vi "PathFinder.vi"(7 "Cost":T3(c390), 8 "TotalCost":u64, 9 "Direction":T1, 11 "AnalysePosition":T2) -> (2 "Directions":T1[](array[typedef]), 3 "Positions":T2[](array[typedef]))   [LabVIEW 2023, in "2024_16.lvclass"]
uses:
  2024_16.lvclass
  Common/AOC_XY(I32).ctl
  Common/AOC_Direction.ctl
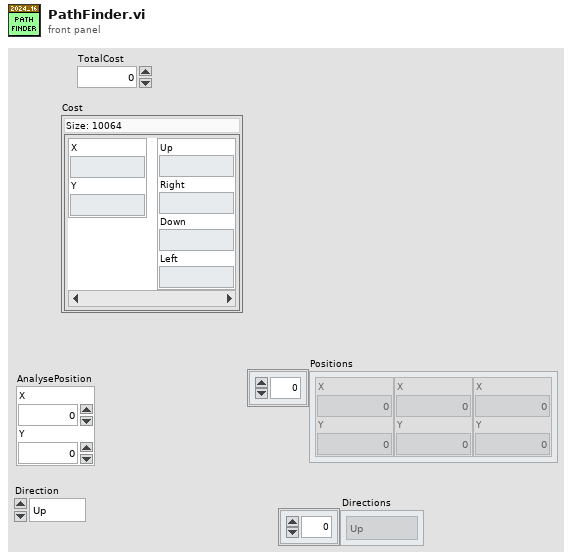
[diagram p1: front panel]
types:
  T1 = typedef "AOC_Direction.ctl" = enum16{"Up", "Right", "Down", "Left"}
  T2 = typedef "AOC_XY(I32).ctl" = cluster{"X":i32, "Y":i32}
  T3 = map{T2, cluster{"Up":u64, "Right":u64, "Down":u64, "Left":u64}}
  T4 = cluster{"Up":u64, "Right":u64, "Down":u64, "Left":u64}
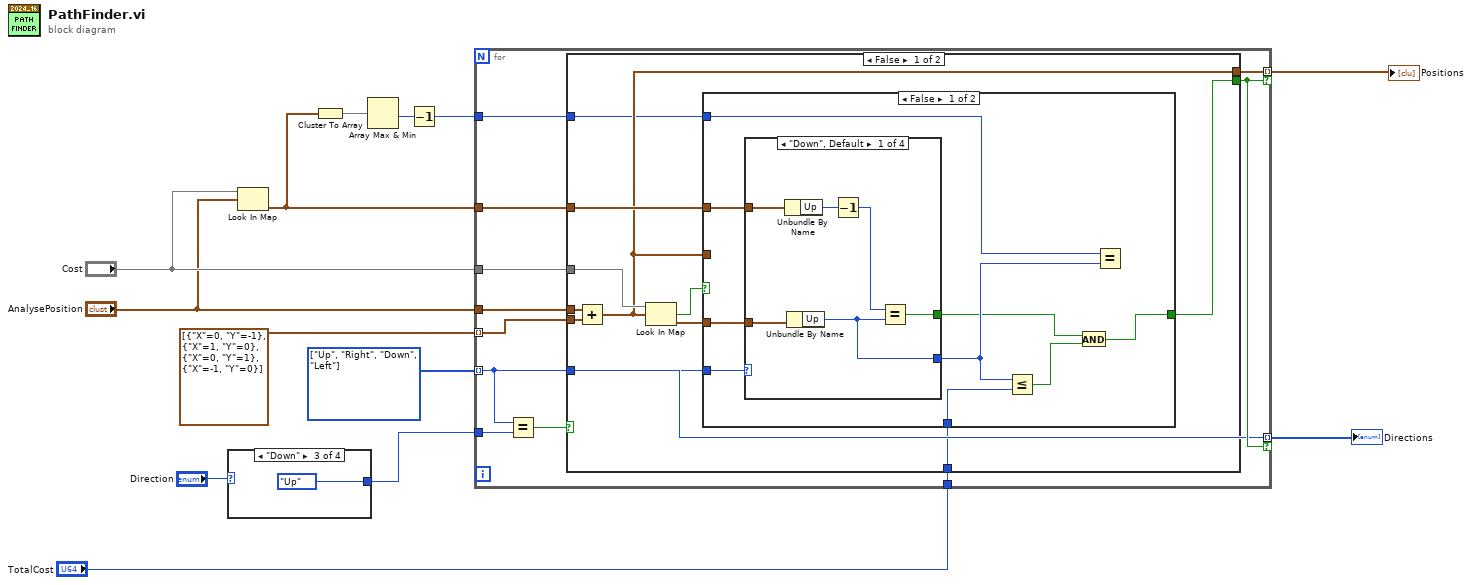
[diagram p0: block diagram]
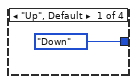
[diagram p2: hidden frame]
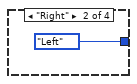
[diagram p3: hidden frame]
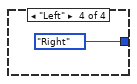
[diagram p4: hidden frame]
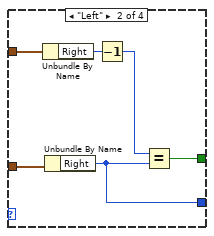
[diagram p5: hidden frame]
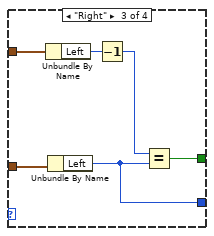
[diagram p6: hidden frame]
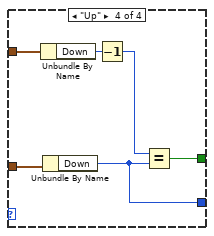
[diagram p7: hidden frame]
diagram:
  w10 = T1[] [enum."Up", enum."Right", enum."Down", enum."Left"] items=["Up", "Right", "Down", "Left"]
  n1 = case shown="\"Down\"" "Direction" {
    tunnel: [AOC_Direction."Down" ("Enum") AOC_Direction."Left" ("Enum") AOC_Direction."Up" ("Enum") AOC_Direction."Right" ("Enum")] -> w6
    frame "Up", Default {
    }
    frame "Right" {
    }
    frame "Down" {
    }
    frame "Left" {
    }
  }
  n2 = Look In Map(map="Cost", key="AnalysePosition") -> (value=w5:T4)  [unwired: 1 in, 1 out]
  n3 = Cluster To Array(cluster=w5) -> (array=w4:u64[])
  n4 = Array Max & Min(array=w4) -> (min value=w3:u64)  [unwired: 3 out]
  n5 = Decrement(x=w3) -> (x-1=w2:u64)
  n6 = for {
    tunnel: cluster{"X":i32, "Y":i32}[] [{"X"=0, "Y"=-1}, {"X"=1, "Y"=0}, {"X"=0, "Y"=1}, {"X"=-1, "Y"=0}] ("Array") -> [w28] mode=indexing
    tunnel: "AnalysePosition" -> [w26]
    tunnel: "Cost" -> [w27]
    tunnel: w10 -> [w22] mode=indexing
    tunnel: w5 -> [w25]
    tunnel: [w24] -> w9 mode=indexing if=w23
    tunnel: [w22] -> w8 mode=indexing if=w23
    tunnel: w6 -> [w21]
    tunnel: w2 -> [w19]
    tunnel: "TotalCost" -> [w18]
    n7 = Equal?(x=w22, y=w21) -> (x = y?=w20:bool)
    n8 = case shown="False" w20 {
      tunnel: w28 -> [w39 _]
      tunnel: w27 -> [w36 _]
      tunnel: w26 -> [w35 _]
      tunnel: w25 -> [w34 _]
      tunnel: [w33 _] -> w24
      tunnel: [w32 _] -> w23
      tunnel: w22 -> [w31 _]
      tunnel: w19 -> [w30 _]
      tunnel: w18 -> [w29 _]
      frame False {
        n9 = Add(x=w35, y=w39) -> (x+y=w33:T2)
        n10 = Look In Map(map=w36, key=w33) -> (key not found?=w38:bool, value=w37:T4)  [unwired: 1 in]
        n11 = case shown="False" w38 {
          tunnel: w37 -> [w46 _]
          tunnel: w33 -> [_ _]
          tunnel: w31 -> [w48 _]
          tunnel: w34 -> [w47 _]
          tunnel: [w40 _] -> w32
          tunnel: w30 -> [w45 _]
          tunnel: w29 -> [w43 _]
          frame False {
            n12 = case shown="\"Down\", Default" w48 {
              tunnel: w47 -> [w54 w60 w66 w72]
              tunnel: w46 -> [w53 w59 w65 w71]
              tunnel: [w50 w56 w62 w68] -> w41
              tunnel: [w49 w55 w61 w67] -> w44
              frame "Down", Default {
                n13 = Unbundle By Name(w54) -> ("Up"=w52:u64)
                n14 = Unbundle By Name(w53) -> ("Up"=w49:u64)
                n15 = Decrement(x=w52) -> (x-1=w51:u64)
                n16 = Equal?(x=w51, y=w49) -> (x = y?=w50:bool)
              }
              frame "Left" {
                n17 = Unbundle By Name(w60) -> ("Right"=w58:u64)
                n18 = Unbundle By Name(w59) -> ("Right"=w55:u64)
                n19 = Decrement(x=w58) -> (x-1=w57:u64)
                n20 = Equal?(x=w57, y=w55) -> (x = y?=w56:bool)
              }
              frame "Right" {
                n21 = Unbundle By Name(w66) -> ("Left"=w64:u64)
                n22 = Unbundle By Name(w65) -> ("Left"=w61:u64)
                n23 = Decrement(x=w64) -> (x-1=w63:u64)
                n24 = Equal?(x=w63, y=w61) -> (x = y?=w62:bool)
              }
              frame "Up" {
                n25 = Unbundle By Name(w72) -> ("Down"=w70:u64)
                n26 = Unbundle By Name(w71) -> ("Down"=w67:u64)
                n27 = Decrement(x=w70) -> (x-1=w69:u64)
                n28 = Equal?(x=w69, y=w67) -> (x = y?=w68:bool)
              }
            }
            n29 = Less Or Equal?(x=w44, y=w43) -> (x <= y?=w42:bool)
            n30 = And(x=w41, y=w42) -> (x .and. y?=w40:bool)
            n31 = Equal?(x=w45, y=w44) -> ()  [unwired: 1 out]
          }
          frame True {
          }
        }
      }
      frame True {
      }
    }
  }
  "Positions" <- w9
  "Directions" <- w8
